vi "StartDataCollection.vi"   [LabVIEW 2010]
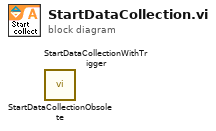
[diagram p0: block diagram]
diagram:
  n1 = call "StartDataCollectionObsolete.vi"() -> ()  [unwired: 10 in, 2 out]
  n2 = call "StartDataCollectionWithTrigger.vi"() -> ()  [unwired: 10 in, 2 out]
